vi "5492_SwitchAutoRight1Cube.vi"(11 "Game Specific Data":string) -> ()   [LabVIEW 2017]
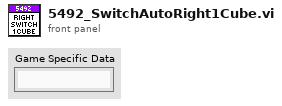
[diagram p1: front panel]
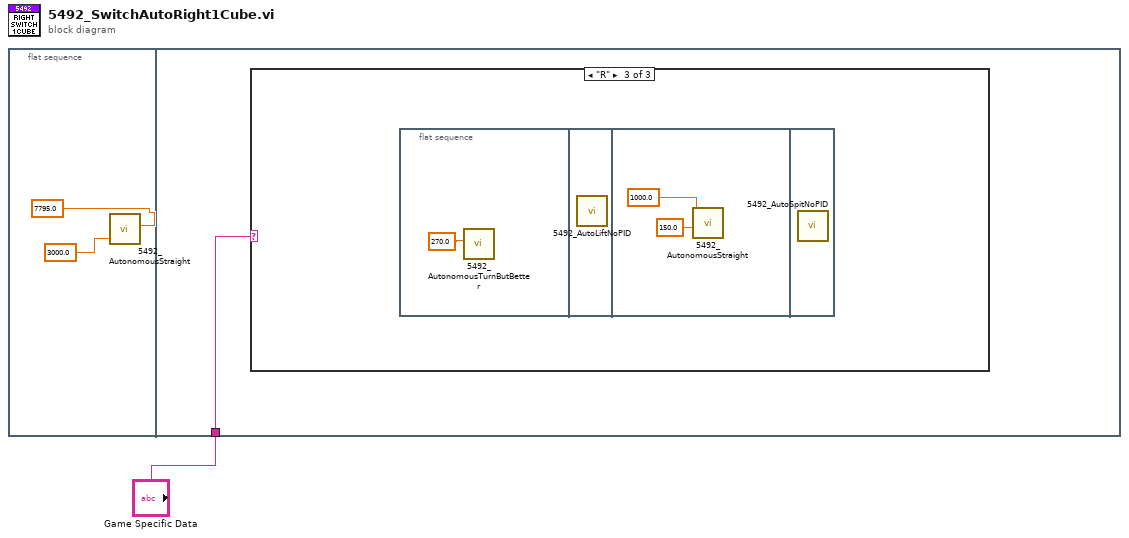
[diagram p0: block diagram]
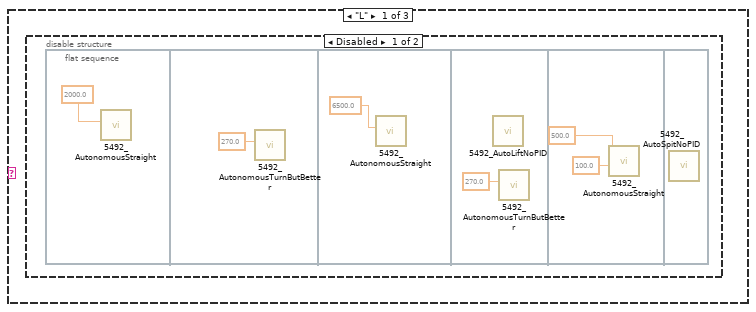
[diagram p2: hidden frame]
diagram:
  n1 = flat-sequence {
    tunnel: "Game Specific Data" -> [w4]
    frame #0 {
      n2 = call "5492_AutonomousStraight.vi"("Length"=3000.0, "Position Goal"=7795.0) -> ()  [unwired: 9 in, 1 out]
    }
    frame #1 {
      n3 = case shown="\"R\"" w4 {
        frame "L" {
          n4 = disable-structure shown="Disabled" {
            frame Disabled {
              n5 = flat-sequence {
                frame #0 {
                  n6 = call "5492_AutonomousStraight.vi"("Position Goal"=2000.0) -> ()  [unwired: 10 in, 1 out]
                }
                frame #1 {
                  n7 = call "5492_AutonomousTurnButBetter.vi"("Yaw Goallll"=270.0) -> ()  [unwired: 10 in, 1 out]
                }
                frame #2 {
                  n8 = call "5492_AutonomousStraight.vi"("Position Goal"=6500.0) -> ()  [unwired: 10 in, 1 out]
                }
                frame #3 {
                  n9 = call "5492_AutoLiftNoPID.vi"() -> ()  [unwired: 12 in]
                  n10 = call "5492_AutonomousTurnButBetter.vi"("Yaw Goallll"=270.0) -> ()  [unwired: 10 in, 1 out]
                }
                frame #4 {
                  n11 = call "5492_AutonomousStraight.vi"("Length"=100.0, "Position Goal"=500.0) -> ()  [unwired: 9 in, 1 out]
                }
                frame #5 {
                  n12 = call "5492_AutoSpitNoPID.vi"() -> ()  [unwired: 12 in]
                }
              }
            }
            frame Enabled {
            }
          }
        }
        frame "como", Default {
        }
        frame "R" {
          n13 = flat-sequence {
            frame #0 {
              n14 = call "5492_AutonomousTurnButBetter.vi"("Yaw Goallll"=270.0) -> ()  [unwired: 10 in, 1 out]
            }
            frame #1 {
              n15 = call "5492_AutoLiftNoPID.vi"() -> ()  [unwired: 12 in]
            }
            frame #2 {
              n16 = call "5492_AutonomousStraight.vi"("Length"=150.0, "Position Goal"=1000.0) -> ()  [unwired: 9 in, 1 out]
            }
            frame #3 {
              n17 = call "5492_AutoSpitNoPID.vi"() -> ()  [unwired: 12 in]
            }
          }
        }
      }
    }
  }
